vi "Get Cluster Element Names.vi"(8 "error in":errorcluster, 11 "LVData":refnum<class "variant.lvclass">) -> (0 "error out":errorcluster, 2 "Element Names":string[](array[string]), 3 "LVData outs":refnum<class "variant.lvclass">)   [LabVIEW 2020, in "variant.lvlib" / "variant.lvclass"]
doc: "Returns the data names of the cluster elements."
uses:
  variant.lvclass
  variant.lvclass/variant.ctl
  Type Descriptor/TD.lvclass
  C:/projects/OpenG-Variant-Data-Library/source/library/Bytes/Bytes.lvclass
  Bytes/Bytes.lvclass/Bytes.ctl
  Bytes/from_byte_array.vi
  Bytes/Bytes.lvclass
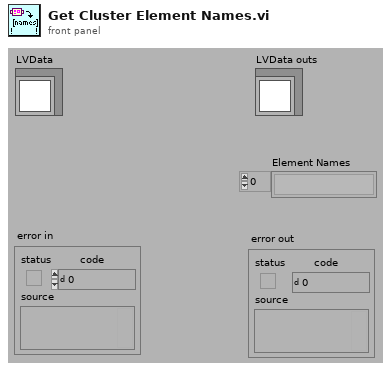
[diagram p1: front panel]
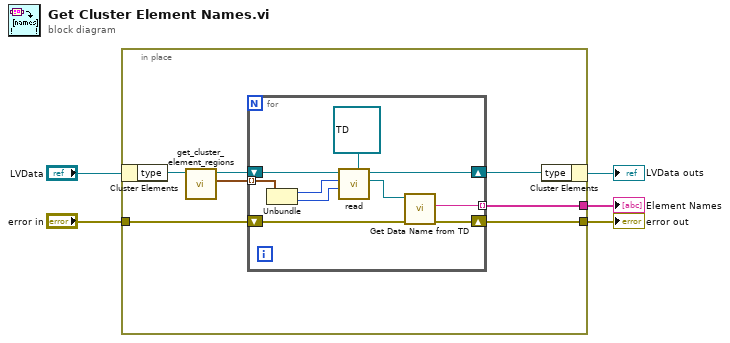
[diagram p0: block diagram]
diagram:
  n1 = in-place {
    in-place-border: [w9] -> w4
    in-place-border: [w7] -> w2
    in-place-border: "error in" -> [w6]
    n2 = in-place-cluster #1("LVData") -> ("type"=w12:refnum<class "TD.lvclass">)
    n3 = call "get_cluster_element_regions.vi"("TypeDescriptor"=w12) -> ("element_regions"=w11:cluster{i32, i32}[], "TypeDescriptor out"=w10:refnum<class "TD.lvclass">)  [unwired: 8 in, 1 out]
    n4 = for {
      tunnel: w11 -> [w22] mode=indexing
      tunnel: [w16] -> w9 mode=indexing
      shift-right: [w15] -> w8
      shift-left: w10 -> [w21]
      shift-right: [w14] -> w7
      shift-left: w6 -> [w13]
      n5 = Unbundle(w22) -> (w20:i32, w19:i32)
      n6 = call "read.vi"("type to read"=refnum<class "TD.lvclass"> refnum ("lvdata.lvlib:TypeDescriptor.lvclass"), "length (-1: rest)"=w19, "offset (-1: current position)"=w20, "Bytes in"=w21) -> ("Bytes read"=w17:refnum<class "TD.lvclass">, "Bytes out"=w15:refnum<class "TD.lvclass">)  [unwired: 6 in]
      n7 = call "Get Data Name from TD.vi"("error in (no error)"=w13, "TypeDescriptor"=w17) -> ("error"=w14:errorcluster, "name"=w16:string)  [unwired: 7 in, 1 out]
    }
    n8 = in-place-cluster #1("type"=w8) -> (→"LVData outs":refnum<class "variant.lvclass">)
  }
  "error out" <- w2
  "Element Names" <- w4
